vi "EmergencyBatteryTemperature (1).vi"(1 "Numeric":dbl) -> (0 "Boolean":bool)   [LabVIEW 2017]
uses:
  EmergencyGLOBAL.vi
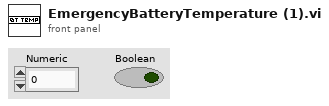
[diagram p1: front panel]
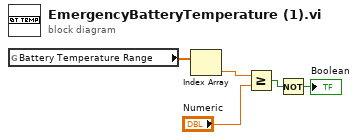
[diagram p0: block diagram]
diagram:
  n1 = global read "EmergencyGLOBAL.vi" "Battery Temperature Range"() -> (w2:dbl[])
  n2 = Index Array(array=w2) -> (element=w3:dbl)  [unwired: 1 in]
  n3 = Greater Or Equal?(x=w3, y="Numeric") -> (x >= y?=w4:bool)
  n4 = Not(x=w4) -> (.not. x?=→"Boolean":bool)
